vi "Destroy All.vi"(8 "error in (no error)":errorcluster, 11 "ONNX Class in":refnum<class "ONNX Class.lvclass">) -> (0 "error out":errorcluster, 3 "ONNX Class out":refnum<class "ONNX Class.lvclass">)   [LabVIEW 2017, in "ONNX Class Library.lvlib" / "ONNX Class.lvclass"]
uses:
  ONNX Class.lvclass
  ONNX Class.lvclass/ONNX Class.ctl
  ONNX Class Library.lvlib
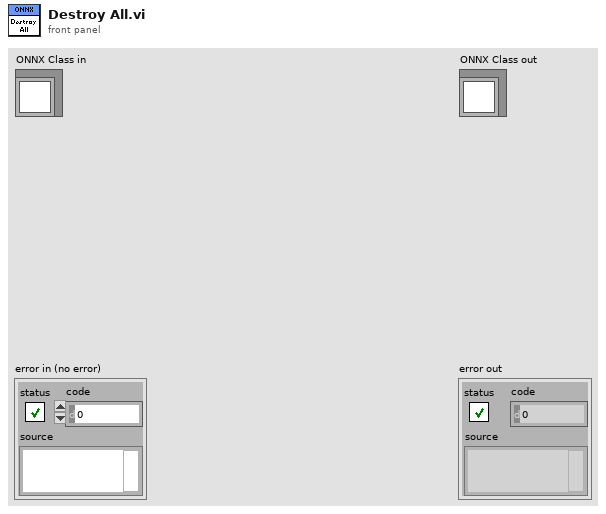
[diagram p1: front panel]
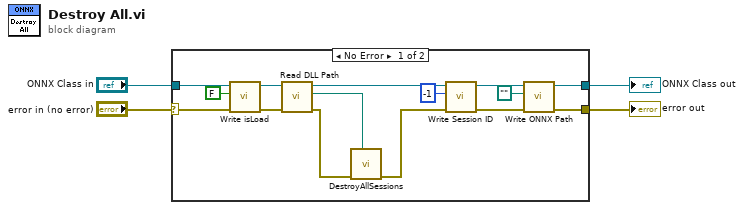
[diagram p0: block diagram]
diagram:
  n1 = case shown="No Error" "error in (no error)" {
    selector: "error in (no error)" -> [w17 w21]
    tunnel: [w12 w21] -> w1
    tunnel: [w14 w20] -> w3
    tunnel: "ONNX Class in" -> [w19 w20]
    frame No Error {
      n2 = call-dynamic "Write isLoad.vi"("error in (no error)"=w17, "isLoad"=FALSE, "ONNX Class in"=w19) -> ("error out"=w5:errorcluster, "ONNX Class out"=w6:refnum<class "ONNX Class.lvclass">)  [unwired: 7 in]
      n3 = call-dynamic "Read DLL Path.vi"("error in (no error)"=w5, "ONNX Class in"=w6) -> ("error out"=w9:errorcluster, "DLL Path"=w7:path, "ONNX Class out"=w16:refnum<class "ONNX Class.lvclass">)  [unwired: 7 in]
      n4 = call "DestroyAllSessions.vi"("DLL path"=w7, "error in (no error)"=w9) -> ("error out"=w8:errorcluster)  [unwired: 9 in]
      n5 = call-dynamic "Write Session ID.vi"("error in (no error)"=w8, "Session ID"=-1, "ONNX Class in"=w16) -> ("error out"=w13:errorcluster, "ONNX Class out"=w15:refnum<class "ONNX Class.lvclass">)  [unwired: 7 in]
      n6 = call-dynamic "Write ONNX Path.vi"("error in (no error)"=w13, "ONNX Path"=path "", "ONNX Class in"=w15) -> ("error out"=w12:errorcluster, "ONNX Class out"=w14:refnum<class "ONNX Class.lvclass">)  [unwired: 7 in]
    }
    frame Error {
    }
  }
  "error out" <- w1
  "ONNX Class out" <- w3
